vi "GEMV_Benchmark(CuLab).vi"() -> ()   [LabVIEW 2020]
doc: "Solves the heat equation in a two-dimensional area using a Finite Element Method."
uses:
  <vilib>/Ngene/CuLab - GPU Accelerated Toolkit/Toolkit/Low_Level/Tensor_Classes/T_Children/T2D/T2D_Children/T2D_SGL/Create_Push.vi
  <vilib>/Ngene/CuLab - GPU Accelerated Toolkit/Toolkit/API/Array/Initialize Array/T1D/CU_Initialize Array_T1D_SGL.vi
  <vilib>/Ngene/CuLab - GPU Accelerated Toolkit/Toolkit/API/Linear Algebra/BLAS2/gemv/CU_gemv/CU_Sgemv.vi
  <vilib>/Ngene/CuLab - GPU Accelerated Toolkit/Toolkit/Low_Level/Tensor_Classes/T_Children/T1D/T1D_Children/T1D_SGL/Pull.vi
  subVIs/Heat Equation Solver.lvlib
  <vilib>/Ngene/CuLab - GPU Accelerated Toolkit/Toolkit/CuLab.lvlib
  <vilib>/ptbypt/NI_PtbyPt.lvlib
  <vilib>/Ngene/CuLab - GPU Accelerated Toolkit/Toolkit/Low_Level/Tensor_Classes/T_Children/T2D/T2D_Children/T2D_SGL/T2D_SGL.lvclass
  <vilib>/Ngene/CuLab - GPU Accelerated Toolkit/Toolkit/Low_Level/Tensor_Classes/T_Children/T1D/T1D_Children/T1D_SGL/T1D_SGL.lvclass
panel:
  out "stop display":bool
  out "Z Graph":sgl[](array[numeric])
  out "time":dbl format="%#_4ps"
  out "Execution Time Graph":dbl(graph)
  out "Error out":errorcluster
  in  "stop":bool
  # "GEMV based on CuLab"
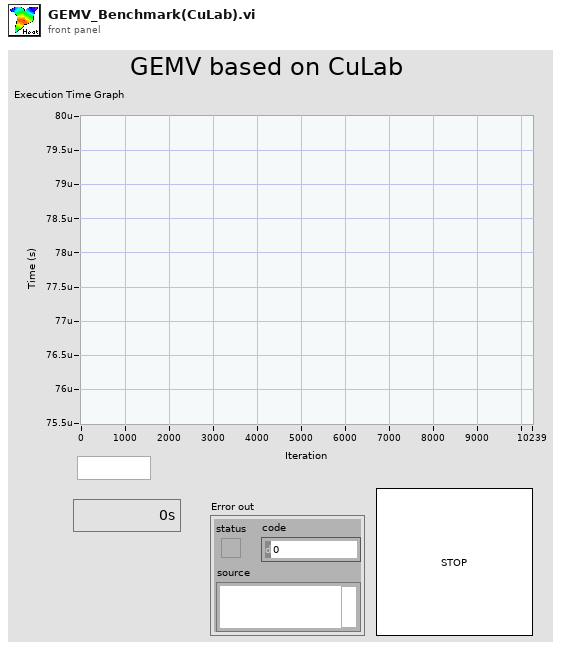
[diagram p1: front panel]
types:
  T1 = typedef "NI_Matrix.lvlib/RealMatrix.ctl" = dbl[][]
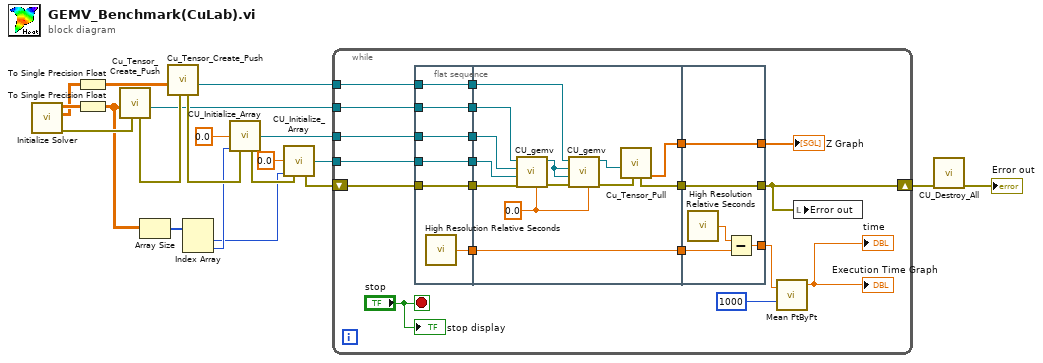
[diagram p0: block diagram]
diagram:
  n1 = call "Initialize Solver.vi"() -> ("error out"=w19:errorcluster, "Mass"=w9:T1, "Stiffness"=w13:T1)  [unwired: 8 in, 1 out]
  n2 = To Single Precision Float(number=w9) -> (single precision float=w7:sgl[][])
  n3 = To Single Precision Float(number=w13) -> (single precision float=w8:sgl[][])
  n4 = call-poly <vilib>:"Cu_Tensor_Create_Push.vi"("error in (no error)"=w19, "CPU_Data_2D_SGL"=w8) -> ("T2D_SGL out"=w15:refnum<class "T2D_SGL.lvclass">, "error out"=w20:errorcluster)  [unwired: 8 in]
  n5 = Array Size(array=w8) -> (size(s)=w12:i32[])
  n6 = call-poly <vilib>:"Cu_Tensor_Create_Push.vi"("error in (no error)"=w20, "CPU_Data_2D_SGL"=w7) -> ("T2D_SGL out"=w14:refnum<class "T2D_SGL.lvclass">, "error out"=w17:errorcluster)  [unwired: 8 in]
  n7 = Index Array(array=w12) -> (element #1=w2:i32, element #2=w10:i32)  [unwired: 2 in]
  n8 = call-poly <vilib>:"CU_Initialize_Array.vi"("element"=sgl 0.0 ("SGL"), "dimension size"=w10, "error in (no error)"=w17) -> ("initialized Tensor"=w11:refnum<class "T1D_SGL.lvclass">, "error out"=w5:errorcluster)  [unwired: 11 in]
  n9 = call-poly <vilib>:"CU_Initialize_Array.vi"("element"=sgl 0.0 ("SGL"), "dimension size"=w2, "error in (no error)"=w5) -> ("initialized Tensor"=w6:refnum<class "T1D_SGL.lvclass">, "error out"=w18:errorcluster)  [unwired: 11 in]
  n10 = while {
    shift-right: [w28] -> w16
    shift-left: w18 -> [w29]
    tunnel: w14 -> [w35]
    tunnel: w15 -> [w34]
    tunnel: w11 -> [w32]
    tunnel: w6 -> [w26]
    stop <- "stop" stop-if-true
    n11 = flat-sequence {
      tunnel: w35 -> [w45]
      tunnel: w34 -> [w46]
      tunnel: [w46] -> w40
      tunnel: [w45] -> w39
      tunnel: [w44] -> w38
      tunnel: [w43] -> w33
      tunnel: w32 -> [w43]
      tunnel: [w42] -> w31
      tunnel: w29 -> [w42]
      tunnel: [w41] -> w27
      tunnel: w26 -> [w41]
      tunnel: w40 -> [w56]
      tunnel: w39 -> [w47]
      tunnel: w38 -> [w58]
      tunnel: [w58] -> w37
      tunnel: w33 -> [w50]
      tunnel: w31 -> [w57]
      tunnel: [w59] -> w30
      tunnel: w27 -> [w53]
      tunnel: [w54] -> w25
      tunnel: w37 -> [w64]
      tunnel: w30 -> [w62]
      tunnel: [w62] -> w28
      tunnel: [w61] -> w21
      tunnel: w25 -> [w61]
      tunnel: [w60] -> w23
      frame #0 {
        n12 = call <vilib>:"High Resolution Relative Seconds.vi"() -> ("relative seconds"=w44:dbl)
      }
      frame #1 {
        w49 = sgl 0.0 ("beta")
        n13 = call-poly <vilib>:"CU_gemv.vi"("beta"=w49, "error in (no error)"=w57, "y"=w53, "x"=w50, "A"=w56) -> ("error out"=w55:errorcluster, "y out"=w48:refnum<class "T1D_SGL.lvclass">)  [unwired: 5 in]
        n14 = call-poly <vilib>:"CU_gemv.vi"("beta"=w49, "error in (no error)"=w55, "y"=w48, "x"=w48, "A"=w47) -> ("error out"=w51:errorcluster, "y out"=w52:refnum<class "T1D_SGL.lvclass">)  [unwired: 5 in]
        n15 = call-poly <vilib>:"Cu_Tensor_Pull.vi"("error in (no error)"=w51, "T1D_SGL in"=w52) -> ("Dest out"=w54:sgl[], "error out"=w59:errorcluster)  [unwired: 7 in, 1 out]
      }
      frame #2 {
        n16 = call <vilib>:"High Resolution Relative Seconds.vi"() -> ("relative seconds"=w63:dbl)
        n17 = Subtract(x=w63, y=w64) -> (x-y=w60:dbl)
      }
    }
    n18 = call <vilib>:"Mean PtByPt.vi"("x"=w23, "sample length"=1000) -> ("mean"=→"Execution Time Graph" →"time":dbl)  [unwired: 2 in, 1 out]
    n19 = local write "Error out"(w28) -> ()
    "Z Graph" <- w21
    "stop display" <- "stop"
  }
  n20 = call <vilib>:"CU_Destroy_All.vi"("error in"=w16) -> ("error out"=→"Error out":errorcluster)  [unwired: 10 in]
